vi "Mathematics_ThresholdAndAlign.vi"(0 "Error In":errorcluster, 1 "Piezo / nm":dbl[](array[numeric]), 2 "Bias In / V":dbl[](array[numeric]), 3 "G/G0":dbl[](array[numeric]), 4 "SAVE?":bool, 5 "On-The-Fly Data Analysis ON":bool, 6 "UP Bound":dbl=0.5, 8 "LOW bound":dbl=-5.0, 9 "Alignment Log(G/G0)":dbl=-0.5, 10 "Femto In / V":dbl[](array[numeric]), 11 "RESET":bool) -> (12 "Femto Out / V":dbl[](array[numeric]), 13 "Enable Histograms?":bool, 14 "Save File?":bool, 15 "Adj. Piezo / nm":dbl[](array[numeric]), 16 "Bias Out / V":dbl[](array[numeric]), 17 "Log(G/G0)":dbl[](array[numeric]), 18 "#saved files":u32, 19 "Error Out":errorcluster)   [LabVIEW 2025]
uses:
  <vilib>/Analysis/baseanly.llb/Mean (DBL).vi
  <vilib>/Analysis/NI_AALBase.lvlib
  <vilib>/ptbypt/NI_PtbyPt.lvlib
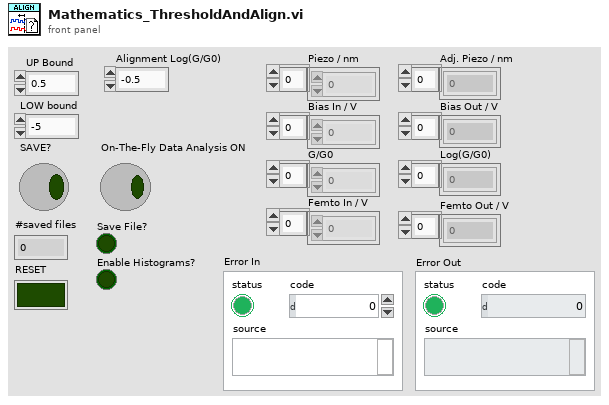
[diagram p1: front panel]
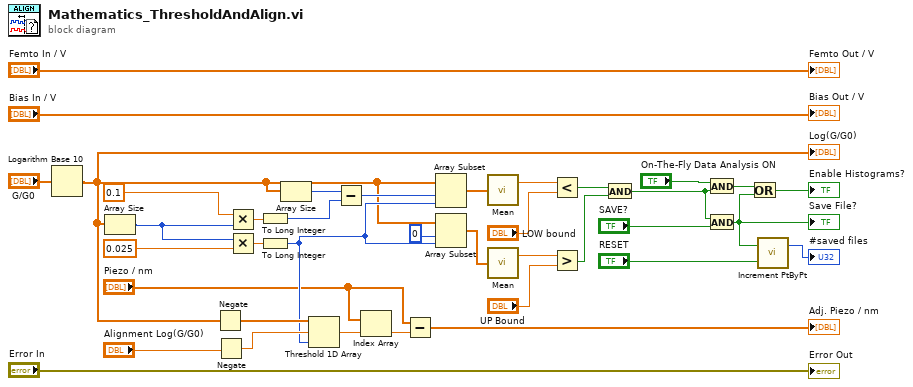
[diagram p0: block diagram]
diagram:
  n1 = Logarithm Base 10(1:"G/G0") -> (0:w3:dbl[])
  "Log(G/G0)" <- w3
  n2 = Array Size(array=w3) -> (size(s)=w2:i32)
  n3 = Negate(x=w3) -> (-x=w13:dbl[])
  n4 = Negate(x="Alignment Log(G/G0)") -> (-x=w11:dbl)
  n5 = Multiply(x=0.1, y=w2) -> (x*y=w17:dbl)
  n6 = Multiply(x=w2, y=0.025) -> (x*y=w16:dbl)
  n7 = To Long Integer(number=w17) -> (32bit integer=w15:i32)
  n8 = To Long Integer(number=w16) -> (32bit integer=w8:i32)
  n9 = Array Size(array=w3) -> (size(s)=w38:i32)
  n10 = Threshold 1D Array(1:w8, 2:w11, 3:w13) -> (0:w9:dbl)
  n11 = Subtract(x=w38, y=w15) -> (x-y=w27:i32)
  n12 = Index Array(array="Piezo / nm", index=w9) -> (element=w10:dbl)
  n13 = Subtract(x="Piezo / nm", y=w10) -> (x-y=→"Adj. Piezo / nm":dbl[])
  n14 = Array Subset(array=w3, index=w27, length=w8) -> (w37:dbl[])
  n15 = Array Subset(array=w3, index=0, length=w8) -> (w36:dbl[])
  n16 = call-poly <vilib>:"Mean.vi"("X"=w37) -> ("mean"=w35:dbl)  [unwired: 1 out]
  n17 = call-poly <vilib>:"Mean.vi"("X"=w36) -> ("mean"=w33:dbl)  [unwired: 1 out]
  n18 = Less?(x=w35, y="LOW bound") -> (x < y?=w31:bool)
  n19 = Greater?(x=w33, y="UP Bound") -> (0:w28:bool)
  n20 = And(x=w31, y=w28) -> (x .and. y?=w24:bool)
  n21 = And(x="On-The-Fly Data Analysis ON", y=w24) -> (x .and. y?=w29:bool)
  n22 = And(x=w24, y="SAVE?") -> (x .and. y?=w21:bool)
  "Save File?" <- w21
  n23 = Or(x=w29, y=w21) -> (x .or. y?=→"Enable Histograms?":bool)
  n24 = call <vilib>:"Increment PtByPt.vi"("initialize"="RESET", "activate"=w21) -> ("counter"=→"#saved files":u32)  [unwired: 1 out]
  "Bias Out / V" <- "Bias In / V"
  "Error Out" <- "Error In"
  "Femto Out / V" <- "Femto In / V"
